vi "Get Data.vi"(8 "error in (no error)":errorcluster, 10 "Data":string, 11 "Serial Devices in":refnum<class "Serial Devices.lvclass">) -> (0 "error out":errorcluster, 3 "Serial Devices out":refnum<class "Serial Devices.lvclass">)   [LabVIEW 2019, in "Serial Devices.lvlib" / "Serial Devices.lvclass"]
uses:
  Serial Devices.lvclass
  Serial Devices.lvclass/Serial Devices.ctl
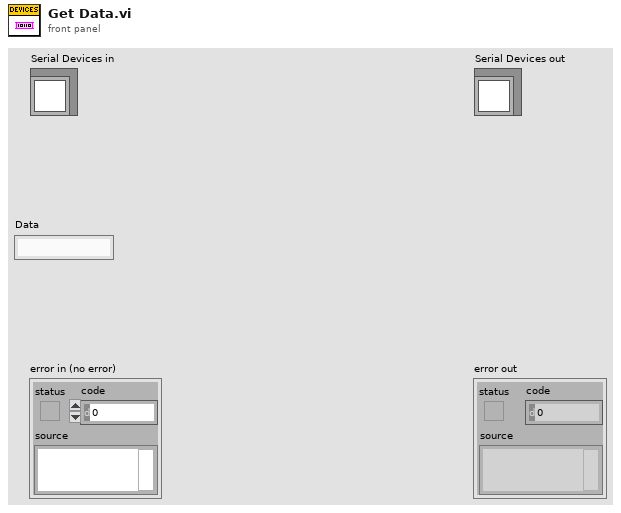
[diagram p1: front panel]
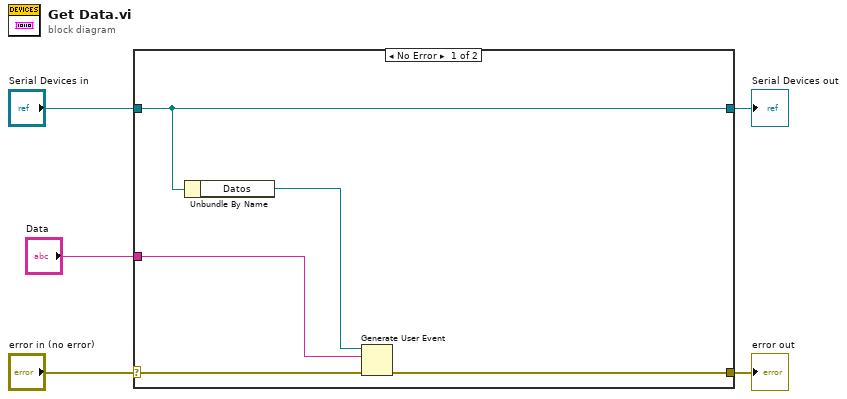
[diagram p0: block diagram]
diagram:
  n1 = case shown="No Error" "error in (no error)" {
    selector: "error in (no error)" -> [w8 w12]
    tunnel: [w6 w12] -> w4
    tunnel: [w10 w11] -> w2
    tunnel: "Serial Devices in" -> [w10 w11]
    tunnel: "Data" -> [w7 _]
    frame No Error {
      n2 = Unbundle By Name(w10) -> ("Datos"=w9:refnum<user-event>)
      n3 = Generate User Event(user event=w9, event data cluster=w7, error in=w8) -> (error out=w6:errorcluster)  [unwired: 1 in, 1 out]
    }
    frame Error {
    }
  }
  "error out" <- w4
  "Serial Devices out" <- w2
